vi "Close.vi"(8 "error in (no error)":errorcluster, 11 "Data.TDMS in":refnum<class "LV-Data.TDMS.lvclass">) -> (0 "error out":errorcluster, 3 "Data.TDMS out":refnum<class "LV-Data.TDMS.lvclass">)   [LabVIEW 2016, in "LV-Data.TDMS.lvclass"]
uses:
  LV-Data.TDMS.lvclass
  LV-Data.TDMS.lvclass/LV-Data.TDMS.ctl
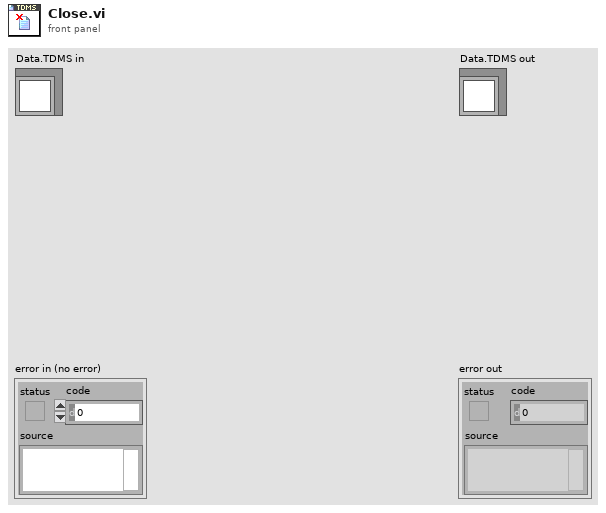
[diagram p1: front panel]
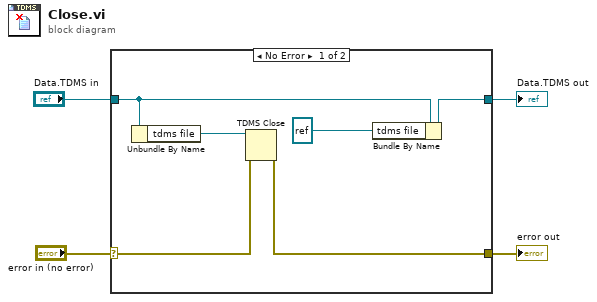
[diagram p0: block diagram]
diagram:
  n1 = case shown="No Error" "error in (no error)" {
    selector: "error in (no error)" -> [w9 w12]
    tunnel: [w5 w11] -> w4
    tunnel: "Data.TDMS in" -> [w6 w11]
    tunnel: [w8 w12] -> w1
    frame No Error {
      n2 = Unbundle By Name(w6) -> ("tdms file"=w10:refnum<k34>)
      n3 = TDMS Close(8:w9, 11:w10) -> (0:w8:errorcluster)  [unwired: 1 out]
      n4 = Bundle By Name(cluster=w6, "tdms file"=refnum<k34> refnum) -> (w5:refnum<class "LV-Data.TDMS.lvclass">)
    }
    frame Error {
    }
  }
  "error out" <- w1
  "Data.TDMS out" <- w4
